vi "Func-엑셀 데이터를 그래프로 출력.vi"() -> ()   [LabVIEW 2015] (continued)
-40\t-39.51\t-24.372\n-40\t-39.51\t-24.377\n-40\t-39.51\t-24.385\n-40\t-39.52\t-24.391\n-40\t-39.52\t-24.396\n-40\t-39.53\t-24.404\n-40\t-39.54\t-24.406\n-40\t-39.54\t-24.41\n-40\t-39.55\t-24.416\n-40\t-39.55\t-24.418\n-40\t-39.56\t-24.424\n-40\t-39.57\t-24.428\n-40\t-39.57\t-24.436\n-40\t-39.58\t-24.442\n-40\t-39.58\t-24.446\n-40\t-39.58\t-24.453\n-40\t-39.58\t-24.456\n-40\t-39.58\t-24.461\n-40\t-39.59\t-24.466\n-40\t-39.59\t-24.471\n-40\t-39.59\t-24.475\n-40\t-39.6\t-24.478\n-40\t-39.6\t-24.486\n-40\t-39.61\t-24.495\n-40\t-39.61\t-24.5\n-40\t-39.62\t-24.504\n-40\t-39.62\t-24.512\n-40\t-39.62\t-24.522\n-40\t-39.63\t-24.521\n-40\t-39.63\t-24.529\n-40\t-39.63\t-24.535\n-40\t-39.63\t-24.539\n-40\t-39.64\t-24.548\n-40\t-39.64\t-24.549\n-40\t-39.64\t-24.556\n-40\t-39.65\t-24.557\n-40\t-39.65\t-24.566\n-40\t-39.65\t-24.573\n-40\t-39.65\t-24.576\n-40\t-39.66\t-24.585\n-40\t-39.66\t-24.593\n-40\t-39.67\t-24.597\n-40\t-39.67\t-24.602\n-40\t-39.68\t-24.609\n-40\t-39.68\t-24.614\n-40\t-39.68\t-24.618\n-40\t-39.69\t-24.62\n-40\t-39.69\t-24.628\n-40\t-39.69\t-24.633\n-40\t-39.7\t-24.636\n-40\t-39.7\t-24.643\n-40\t-39.71\t-24.652\n-40\t-39.71\t-24.66\n-40\t-39.71\t-24.667\n-40\t-39.71\t-24.672\n-40\t-39.71\t-24.676\n-40\t-39.72\t-24.682\n-40\t-39.72\t-24.684\n-40\t-39.72\t-24.687\n-40\t-39.72\t-24.691\n-40\t-39.72\t-24.693\n-40\t-39.72\t-24.699\n-40\t-39.72\t-24.705\n-40\t-39.72\t-24.714\n-40\t-39.73\t-24.719\n-40\t-39.73\t-24.729\n-40\t-39.73\t-24.737\n-40\t-39.73\t-24.744\n-40\t-39.74\t-24.747\n-40\t-39.74\t-24.753\n-40\t-39.74\t-24.76\n-40\t-39.74\t-24.764\n-40\t-39.74\t-24.769\n-40\t-39.74\t-24.772\n-40\t-39.74\t-24.78\n-40\t-39.75\t-24.784\n-40\t-39.75\t-24.787\n-40\t-39.75\t-24.795\n-40\t-39.75\t-24.796\n-40\t-39.76\t-24.802\n-40\t-39.76\t-24.807\n-40\t-39.76\t-24.812\n-40\t-39.76\t-24.818\n-40\t-39.76\t-24.822\n-40\t-39.76\t-24.828\n-40\t-39.77\t-24.832\n-40\t-39.77\t-24.839\n-40\t-39.78\t-24.842\n-40\t-39.78\t-24.845\n-40\t-39.78\t-24.857\n-40\t-39.78\t-24.864\n-40\t-39.79\t-24.87\n-40\t-39.79\t-24.879\n-40\t-39.79\t-24.888\n-40\t-39.79\t-24.893\n-40\t-39.8\t-24.896\n-40\t-39.8\t-24.9\n-40\t-39.8\t-24.903\n-40\t-39.8\t-24.908\n-40\t-39.81\t-24.909\n-40\t-39.81\t-24.915\n-40\t-39.81\t-24.923\n-40\t-39.81\t-24.926\n-40\t-39.81\t-24.93\n-40\t-39.81\t-24.937\n-40\t-39.81\t-24.944\n-40\t-39.81\t-24.948\n-40\t-39.82\t-24.954\n-40\t-39.82\t-24.962\n-40\t-39.82\t-24.967\n-40\t-39.83\t-24.972\n-40\t-39.83\t-24.974\n-40\t-39.83\t-24.979\n-40\t-39.83\t-24.985\n-40\t-39.84\t-24.986\n-40\t-39.84\t-24.995\n-40\t-39.84\t-25.003\n-40\t-39.84\t-25.011\n-40\t-39.84\t-25.014\n-40\t-39.85\t-25.022\n-40\t-39.85\t-25.029\n-40\t-39.85\t-25.031\n-40\t-39.86\t-25.034\n-40\t-39.86\t-25.039\n-40\t-39.86\t-25.044\n-40\t-39.86\t-25.049\n-40\t-39.87\t-25.054\n-40\t-39.87\t-25.059\n-40\t-39.87\t-25.067\n-40\t-39.87\t-25.069\n-40\t-39.88\t-25.077\n-40\t-39.88\t-25.082\n-40\t-39.88\t-25.088\n-40\t-39.88\t-25.093\n-40\t-39.88\t-25.1\n-40\t-39.88\t-25.106\n-40\t-39.88\t-25.11\n-40\t-39.88\t-25.116\n-40\t-39.88\t-25.121\n-40\t-39.88\t-25.126\n-40\t-39.88\t-25.134\n-40\t-39.88\t-25.138\n-40\t-39.89\t-25.145\n-40\t-39.89\t-25.154\n-40\t-39.89\t-25.161\n-40\t-39.89\t-25.163\n-40\t-39.9\t-25.168\n-40\t-39.9\t-25.172\n-40\t-39.9\t-25.176\n-40\t-39.9\t-25.181\n-40\t-39.9\t-25.186\n-40\t-39.9\t-25.194\n-40\t-39.91\t-25.2\n-40\t-39.91\t-25.207\n-40\t-39.92\t-25.212\n-40\t-39.92\t-25.219\n-40\t-39.92\t-25.223\n-40\t-39.92\t-25.227\n-40\t-39.93\t-25.236\n-40\t-39.93\t-25.239\n-40\t-39.93\t-25.246\n-40\t-39.93\t-25.253\n-40\t-39.93\t-25.258\n-40\t-39.94\t-25.263\n-40\t-39.94\t-25.267\n-40\t-39.94\t-25.274\n-40\t-39.95\t-25.279\n-40\t-39.95\t-25.285\n-40\t-39.95\t-25.29\n-40\t-39.95\t-25.295\n-40\t-39.95\t-25.3\n-40\t-39.95\t-25.305\n-40\t-39.95\t-25.311\n-40\t-39.95\t-25.316\n-40\t-39.96\t-25.32\n-40\t-39.96\t-25.321\n-40\t-39.96\t-25.326\n-40\t-39.97\t-25.328\n-40\t-39.97\t-25.331\n-40\t-39.97\t-25.338\n-40\t-39.97\t-25.344\n-40\t-39.97\t-25.35\n-40\t-39.97\t-25.36\n-40\t-39.97\t-25.363\n-40\t-39.98\t-25.364\n-40\t-39.98\t-25.367\n-40\t-39.98\t-25.37\n-40\t-39.98\t-25.373\n-40\t-39.98\t-25.379\n-40\t-39.98\t-25.389\n-40\t-39.98\t-25.398\n-40\t-39.98\t-25.408\n-40\t-39.98\t-25.413\n-40\t-39.99\t-25.418\n-40\t-39.99\t-25.424\n-40\t-40\t-25.425\n-40\t-40\t-25.428\n-40\t-40\t-25.432\n-40\t-40\t-25.437\n-40\t-40\t-25.445\n-40\t-40\t-25.453\n-40\t-40\t-25.458\n-40\t-40\t-25.461\n-40\t-40\t-25.47\n-40\t-40\t-25.477\n-40\t-40\t-25.48\n-40\t-40\t-25.486\n-40\t-40\t-25.492\n-40\t-40\t-25.498\n-40\t-40\t-25.501\n-40\t-40\t-25.504\n-40\t-40\t-25.507\n-40\t-40\t-25.509\n-40\t-40\t-25.512\n-40\t-40\t-25.517\n-40\t-40\t-25.522\n-40\t-40\t-25.525\n-40\t-40\t-25.53\n-40\t-40\t-25.539\n-40\t-40\t-25.545\n-40\t-40\t-25.549\n-40\t-40\t-25.557\n-40\t-40\t-25.563\n-40\t-40\t-25.568\n-40\t-40\t-25.572\n-40\t-40\t-25.579\n-40\t-40\t-25.583\n-40\t-40\t-25.589\n-40\t-40\t-25.594\n-40\t-40\t-25.596\n-40\t-40\t-25.603\n-40\t-40\t-25.605\n-40\t-40\t-25.61\n-40\t-40\t-25.618\n-40\t-40\t-25.62\n-40\t-40\t-25.626\n-40\t-40\t-25.631\n-40\t-40\t-25.638\n-40\t-40\t-25.645\n-40\t-40\t-25.648\n-40\t-40\t-25.655\n-40\t-40\t-25.661\n-40\t-40\t-25.667\n-40\t-40\t-25.671\n-40\t-40\t-25.677\n-40\t-40\t-25.682\n-40\t-40\t-25.687\n-40\t-40\t-25.691\n-40\t-40\t-25.697\n-40\t-40\t-25.698\n-40\t-40\t-25.704\n-40\t-40\t-25.707\n-40\t-40\t-25.711\n-40\t-40\t-25.716\n-40\t-40\t-25.723\n-40\t-40\t-25.731\n-40\t-40\t-25.736\n-40\t-40\t-25.742\n-40\t-40\t-25.746\n-40\t-40\t-25.749\n-40\t-40\t-25.754\n-40\t-40\t-25.758\n-40\t-40\t-25.764\n-40\t-40\t-25.769\n-40\t-40\t-25.775\n-40\t-40\t-25.784\n-40\t-40\t-25.791\n-40\t-40\t-25.793\n-40\t-40.02\t-25.802\n-40\t-40.02\t-25.808\n-40\t-40.02\t-25.814\n-40\t-40.02\t-25.816\n-40\t-40.02\t-25.82\n-40\t-40.02\t-25.825\n-40\t-40.02\t-25.828\n-40\t-40.02\t-25.835\n-40\t-40.02\t-25.837\n-40\t-40.02\t-25.846\n-40\t-40.02\t-25.85\n-40\t-40.02\t-25.854\n-40\t-40.02\t-25.865\n-40\t-40.02\t-25.867\n-40\t-40.02\t-25.867\n-40\t-40.02\t-25.873\n-40\t-40.02\t-25.879\n-40\t-40.02\t-25.885\n-40\t-40.02\t-25.887\n-40\t-40.02\t-25.891\n-40\t-40.02\t-25.898\n-40\t-40.02\t-25.902\n-40\t-40.02\t-25.904\n-40\t-40.02\t-25.904\n-40\t-40.02\t-25.912\n-40\t-40.02\t-25.916\n-40\t-40.02\t-25.92\n-40\t-40.02\t-25.927\n-40\t-40.02\t-25.934\n-40\t-40.02\t-25.942\n-40\t-40.02\t-25.949\n-40\t-40.02\t-25.951\n-40\t-40.02\t-25.952\n-40\t-40.02\t-25.956\n-40\t-40.02\t-25.961\n-40\t-40.02\t-25.963\n-40\t-40.02\t-25.965\n-40\t-40.02\t-25.972\n-40\t-40.02\t-25.982\n-40\t-40.02\t-25.99\n-40\t-40.02\t-25.993\n-40\t-40.02\t-25.997\n-40\t-40.02\t-26.003\n-40\t-40.02\t-26.008\n-40\t-40.02\t-26.016\n-40\t-40.02\t-26.021\n-40\t-40.02\t-26.029\n-40\t-40.02\t-26.034\n-40\t-40.02\t-26.039\n-40\t-40.02\t-26.043\n-40\t-40.02\t-26.042\n-40\t-40.02\t-26.049\n-40\t-40.02\t-26.05\n-40\t-40.02\t-26.053\n-40\t-40.02\t-26.062\n-40\t-40.02\t-26.067\n-40\t-40.02\t-26.072\n-40\t-40.02\t-26.075\n-40\t-40.02\t-26.079\n-40\t-40.02\t-26.083\n-40\t-40.02\t-26.089\n-40\t-40.02\t-26.093\n-40\t-40.02\t-26.098\n-40\t-40.02\t-26.106\n-40\t-40.02\t-26.109\n-40\t-40.02\t-26.117\n-40\t-40.02\t-26.123\n-40\t-40.02\t-26.126\n-40\t-40.02\t-26.13\n-40\t-40.02\t-26.135\n-40\t-40.02\t-26.14\n-40\t-40.02\t-26.142\n-40\t-40.03\t-26.145\n-40\t-40.03\t-26.152\n-40\t-40.03\t-26.157\n-40\t-40.03\t-26.163\n-40\t-40.03\t-26.167\n-40\t-40.03\t-26.173\n-40\t-40.03\t-26.181\n-40\t-40.03\t-26.184\n-40\t-40.03\t-26.188\n-40\t-40.03\t-26.192\n-40\t-40.03\t-26.194\n-40\t-40.03\t-26.195\n-40\t-40.03\t-26.202\n-40\t-40.02\t-26.207\n-40\t-40.02\t-26.211\n-40\t-40.02\t-26.219\n-40\t-40.02\t-26.227\n-40\t-40.02\t-26.231\n-40\t-40.02\t-26.236\n-40\t-40.02\t-26.239\n-40\t-40.02\t-26.242\n-40\t-40.02\t-26.248\n-40\t-40.02\t-26.25\n-40\t-40.02\t-26.256\n-40\t-40.02\t-26.266\n-40\t-40.02\t-26.271\n-40\t-40.02\t-26.277\n-40\t-40.02\t-26.28\n-40\t-40.02\t-26.286\n-40\t-40.02\t-26.29\n-40\t-40.02\t-26.292\n-40\t-40.02\t-26.295\n-40\t-40.02\t-26.298\n-40\t-40.02\t-26.307\n-40\t-40.02\t-26.312\n-40\t-40.02\t-26.32\n-40\t-40.02\t-26.327\n-40\t-40.02\t-26.334\n-40\t-40.03\t-26.337\n-40\t-40.03\t-26.343\n-40\t-40.03\t-26.347\n-40\t-40.03\t-26.349\n-40\t-40.03\t-26.354\n-40\t-40.03\t-26.356\n-40\t-40.03\t-26.362\n-40\t-40.03\t-26.368\n-40\t-40.03\t-26.371\n-40\t-40.03\t-26.375\n-40\t-40.03\t-26.381\n-40\t-40.03\t-26.387\n-40\t-40.03\t-26.39\n-40\t-40.03\t-26.396\n-40\t-40.03\t-26.402\n-40\t-40.02\t-26.407\n-40\t-40.02\t-26.41\n-40\t-40.02\t-26.413\n-40\t-40.02\t-26.418\n-40\t-40.02\t-26.42\n-40\t-40.02\t-26.423\n-40\t-40.02\t-26.426\n-40\t-40.02\t-26.436\n-40\t-40.02\t-26.439\n-40\t-40.02\t-26.445\n-40\t-40.02\t-26.453\n-40\t-40.02\t-26.455\n-40\t-40.02\t-26.46\n-40\t-40.02\t-26.461\n-40\t-40.02\t-26.469\n-40\t-40.02\t-26.47\n-40\t-40.02\t-26.477\n-40\t-40.02\t-26.482\n-40\t-40.02\t-26.49\n-40\t-40.02\t-26.497\n-40\t-40.02\t-26.5\n-40\t-40.02\t-26.506\n-40\t-40.02\t-26.511\n-40\t-40.02\t-26.52\n-40\t-40.02\t-26.521\n-40\t-40.02\t-26.527\n-40\t-40.02\t-26.532\n-40\t-40.02\t-26.536\n-40\t-40.02\t-26.538\n-40\t-40.02\t-26.542\n-40\t-40.02\t-26.546\n-40\t-40.02\t-26.555\n-40\t-40.02\t-26.558\n-40\t-40.02\t-26.564\n-40\t-40.02\t-26.57\n-40\t-40.02\t-26.573\n-40\t-40.02\t-26.578\n-40\t-40.02\t-26.582\n-40\t-40.02\t-26.584\n-40\t-40.02\t-26.588\n-40\t-40.02\t-26.594\n-40\t-40.02\t-26.595\n-40\t-40.02\t-26.594\n-40\t-40.02\t-26.598\n-40\t-40.02\t-26.607\n-40\t-40.02\t-26.609\n-40\t-40.02\t-26.613\n-40\t-40.02\t-26.62\n-40\t-40.02\t-26.627\n-40\t-40.02\t-26.63\n-40\t-40.02\t-26.634\n-40\t-40.02\t-26.637\n-40\t-40.02\t-26.645\n-40\t-40.02\t-26.646\n-40\t-40.02\t-26.651\n-40\t-40.02\t-26.658\n-40\t-40.02\t-26.66\n-40\t-40.02\t-26.664\n-40\t-40\t-26.67\n-40\t-40\t-26.675\n-40\t-40\t-26.677\n-40\t-40\t-26.684\n-40\t-40\t-26.687\n-40\t-40\t-26.693\n-40\t-40\t-26.696\n-40\t-40\t-26.7\n-40\t-40\t-26.708\n-40\t-40\t-26.711\n-40\t-40\t-26.713\n-40\t-40\t-26.716\n-40\t-40.02\t-26.72\n-40\t-40\t-26.725\n-40\t-40\t-26.725\n-40\t-40\t-26.732\n-40\t-40\t-26.739\n-40\t-40\t-26.743\n-40\t-40.02\t-26.751\n-40\t-40.02\t-26.755\n-40\t-40.02\t-26.763\n-40\t-40.02\t-26.768\n-40\t-40.02\t-26.771\n-40\t-40\t-26.774\n-40\t-40.02\t-26.776\n-40\t-40.02\t-26.78\n-40\t-40.02\t-26.782\n-40\t-40.02\t-26.786\n-40\t-40.02\t-26.789\n-40\t-40.02\t-26.795\n-40\t-40.02\t-26.801\n-40\t-40.02\t-26.802\n-40\t-40.02\t-26.805\n-40\t-40.02\t-26.808\n-40\t-40.02\t-26.811\n-40\t-40.02\t-26.815\n-40\t-40.02\t-26.823\n-40\t-40.02\t-26.829\n-40\t-40.02\t-26.833\n-40\t-40.02\t-26.84\n-40\t-40.02\t-26.848\n-40\t-40.02\t-26.847\n-40\t-40.02\t-26.852\n-40\t-40.02\t-26.856\n-40\t-40.02\t-26.861\n-40\t-40.02\t-26.863\n-40\t-40.02\t-26.866\n-40\t-40.02\t-26.873\n-40\t-40.02\t-26.88\n-40\t-40.02\t-26.883\n-40\t-40.02\t-26.888\n-40\t-40.02\t-26.891\n-40\t-40.02\t-26.894\n-40\t-40.02\t-26.899\n-40\t-40.02\t-26.9\n-40\t-40.02\t-26.903\n-40\t-40.02\t-26.909\n-40\t-40.02\t-26.914\n-40\t-40.02\t-26.918\n-40\t-40.02\t-26.924\n-40\t-40.02\t-26.929\n-40\t-40.02\t-26.932\n-40\t-40.02\t-26.938\n-40\t-40.02\t-26.944\n-40\t-40.02\t-26.946\n-40\t-40.02\t-26.949\n-40\t-40.02\t-26.95\n-40\t-40.02\t-26.955\n-40\t-40.02\t-26.958\n-40\t-40.02\t-26.959\n-40\t-40.02\t-26.965\n-40\t-40.02\t-26.971\n-40\t-40.02\t-26.977\n-40\t-40.02\t-26.983\n-40\t-40.02\t-26.99\n-40\t-40.02\t-26.993\n-40\t-40.02\t-26.996\n-40\t-40.02\t-27.003\n-40\t-40.02\t-27.006\n-40\t-40.02\t-27.011\n-40\t-40.02\t-27.013\n-40\t-40.02\t-27.017\n-40\t-40.02\t-27.019\n-40\t-40.02\t-27.025\n-40\t-40.02\t-27.028\n-40\t-40.02\t-27.027\n-40\t-40.02\t-27.03\n-40\t-40.02\t-27.036\n-40\t-40.02\t-27.041\n-40\t-40.02\t-27.041\n-40\t-40.02\t-27.046\n-40\t-40.02\t-27.052\n-40\t-40.02\t-27.062\n-40\t-40.02\t-27.063\n-40\t-40.02\t-27.068\n-40\t-40.02\t-27.077\n-40\t-40.02\t-27.08\n-40\t-40.02\t-27.084\n-40\t-40.02\t-27.083\n-40\t-40.02\t-27.084\n-40\t-40.02\t-27.085\n-40\t-40.02\t-27.092\n-40\t-40.02\t-27.096\n-40\t-40.02\t-27.096\n-40\t-40.02\t-27.103\n-40\t-40.02\t-27.112\n-40\t-40.02\t-27.118\n-40\t-40.02\t-27.121\n-40\t-40.02\t-27.127\n-40\t-40.02\t-27.131\n-40\t-40.02\t-27.137\n-40\t-40.02\t-27.139\n-40\t-40.02\t-27.141\n-40\t-40.02\t-27.143\n-40\t-40.02\t-27.144\n-40\t-40.02\t-27.147\n-40\t-40.02\t-27.153\n-40\t-40.02\t-27.157\n-40\t-40.02\t-27.158\n-40\t-40.02\t-27.166\n-40\t-40.02\t-27.171\n-40\t-40.02\t-27.172\n-40\t-40.02\t-27.174\n-40\t-40.02\t-27.176\n-40\t-40.02\t-27.181\n-40\t-40.02\t-27.187\n-40\t-40.02\t-27.187\n-40\t-40.02\t-27.193\n-40\t-40.02\t-27.198\n-40\t-40.02\t-27.2\n-40\t-40\t-27.205\n-40\t-40\t-27.209\n-40\t-40\t-27.216\n-40\t-40\t-27.221\n-40\t-40\t-27.226\n-40\t-40\t-27.229\n-40\t-40\t-27.23\n-40\t-40\t-27.233\n-40\t-40\t-27.234\n-40\t-40\t-27.238\n-40\t-40\t-27.245\n-40\t-40\t-27.25\n-40\t-40\t-27.254\n-40\t-40\t-27.261\n-40\t-40\t-27.264\n-40\t-40\t-27.267\n-40\t-40\t-27.268\n-40\t-40\t-27.272\n-40\t-40\t-27.277\n-40\t-40\t-27.28\n-40\t-40\t-27.283\n-40\t-40\t-27.287\n-40\t-40\t-27.29\n-40\t-40\t-27.291\n-40\t-40\t-27.296\n-40\t-40\t-27.3\n-40\t-40\t-27.305\n-40\t-40\t-27.309\n-40\t-40\t-27.316\n-40\t-40\t-27.321\n-40\t-40\t-27.321\n-40\t-40\t-27.321\n-40\t-40\t-27.322\n-40\t-40\t-27.327\n-40\t-40\t-27.329\n-40\t-40\t-27.333\n-40\t-40\t-27.339\n-40\t-40\t-27.348\n-40\t-40\t-27.352\n-40\t-40\t-27.355\n-40\t-40\t-27.358\n-40\t-40\t-27.361\n-40\t-40\t-27.364\n-40\t-40\t-27.368\n-40\t-40\t-27.37\n-40\t-40\t-27.371\n-40\t-40\t-27.379\n-40\t-40\t-27.382\n-40\t-40\t-27.384\n-40\t-40\t-27.387\n-40\t-40\t-27.393\n-40\t-40\t-27.394\n-40\t-40\t-27.395\n-40\t-40\t-27.398\n-40\t-40\t-27.401\n-40\t-40\t-27.406\n-40\t-40\t-27.409\n-40\t-40\t-27.415\n-40\t-40\t-27.418\n-40\t-40\t-27.42\n-40\t-40\t-27.425\n-40\t-40\t-27.429\n-40\t-40\t-27.432\n-40\t-40\t-27.437\n-40\t-40\t-27.445\n-40\t-40\t-27.451\n-40\t-40\t-27.454\n-40\t-40\t-27.454\n-40\t-40\t-27.455\n-40\t-40\t-27.457\n-40\t-40\t-27.461\n-40\t-40\t-27.462\n-40\t-40\t-27.465\n-40\t-40\t-27.474\n-40\t-40\t-27.478\n-40\t-40\t-27.484\n-40\t-40\t-27.491\n-40\t-40\t-27.494\n-40\t-40\t-27.499\n-40\t-40\t-27.5\n-40\t-40\t-27.501\n-40\t-40\t-27.502\n-40\t-40\t-27.503\n-40\t-40\t-27.506\n-40\t-40\t-27.507\n-40\t-40\t-27.508\n-40\t-40\t-27.512\n-40\t-40\t-27.515\n-40\t-40\t-27.521\n-40\t-40\t-27.523\n-40\t-40\t-27.527\n-40\t-40\t-27.539\n-40\t-40\t-27.545\n-40\t-40\t-27.549\n-40\t-40\t-27.551\n-40\t-40\t-27.556\n-40\t-40\t-27.561\n-40\t-40\t-27.563\n-40\t-40\t-27.567\n-40\t-40\t-27.571\n-40\t-40\t-27.572\n-40\t-40\t-27.575\n-40\t-40\t-27.58\n-40\t-40\t-27.585\n-40\t-40\t-27.587\n-40\t-40\t-27.588\n-40\t-40\t-27.593\n-40\t-40\t-27.595\n-40\t-40\t-27.595\n-40\t-40\t-27.598\n-40\t-40\t-27.602\n-40\t-40\t-27.608\n-40\t-40\t-27.612\n-40\t-40\t-27.616\n-40\t-40\t-27.619\n-40\t-40\t-27.624\n-40\t-40\t-27.627\n-40\t-40\t-27.629\n-40\t-40\t-27.634\n-40\t-40\t-27.636\n-40\t-40\t-27.636\n-40\t-40\t-27.641\n-40\t-40\t-27.647\n-40\t-40\t-27.65\n-40\t-40\t-27.655\n-40\t-40\t-27.656\n-40\t-40\t-27.66\n-40\t-40\t-27.661\n-40\t-40\t-27.657\n-40\t-40\t-27.658\n-40\t-40\t-27.664\n-40\t-40\t-27.67\n-40\t-40\t-27.675\n-40\t-40\t-27.677\n-40\t-40\t-27.681\n-40\t-40\t-27.687\n-40\t-40\t-27.686\n-40\t-40\t-27.686\n-40\t-40\t-27.689\n-40\t-40\t-27.693\n-40\t-40\t-27.697\n-40\t-40\t-27.701\n-40\t-40\t-27.708\n-40\t-40\t-27.712\n-40\t-40\t-27.714\n-40\t-40\t-27.721\n-40\t-40\t-27.725\n-40\t-40\t-27.726\n-40\t-40\t-27.727\n-40\t-40\t-27.731\n-40\t-40\t-27.73\n-40\t-40\t-27.73\n-40\t-40\t-27.736\n-40\t-40\t-27.736\n-40\t-40\t-27.745\n-40\t-40\t-27.748\n-40\t-40\t-27.753\n-40\t-40\t-27.761\n-40\t-40\t-27.761\n-40\t-40\t-27.766\n-40\t-40\t-27.765\n-40\t-40\t-27.77\n-40\t-40\t-27.773\n-40\t-40\t-27.779\n-40\t-40\t-27.782\n-40\t-40\t-27.783\n-40\t-40\t-27.789\n-40\t-40\t-27.791\n-40\t-40\t-27.792\n-40\t-40\t-27.793\n-40\t-40\t-27.796\n-40\t-40\t-27.803\n-40\t-40\t-27.806\n-40\t-40\t-27.809\n-40\t-40\t-27.816\n-40\t-40\t-27.82\n-40\t-40\t-27.822\n-40\t-40\t-27.824\n-40\t-40\t-27.827\n-40\t-40\t-27.83\n-40\t-40\t-27.832\n-40\t-40\t-27.834\n-40\t-40\t-27.837\n-40\t-40\t-27.84\n-40\t-40\t-27.845\n-40\t-40\t-27.846\n-40\t-40\t-27.849\n-40\t-40\t-27.852\n-40\t-40\t-27.854\n-40\t-40\t-27.855\n-40\t-40\t-27.857\n-40\t-40\t-27.864\n-40\t-40\t-27.869\n-40\t-40\t-27.87\n-40\t-40\t-27.871\n-40\t-40\t-27.876\n-40\t-40\t-27.879\n-40\t-40\t-27.879\n-40\t-40\t-27.88\n-40\t-40\t-27.884\n-40\t-40\t-27.887\n-40\t-40\t-27.893\n-40\t-40\t-27.896\n-40\t-40\t-27.9\n-40\t-40\t-27.905\n-40\t-40\t-27.904\n-40\t-40\t-27.909\n-40\t-40\t-27.909\n-40\t-40\t-27.908\n-40\t-40\t-27.909\n-40\t-40\t-27.91\n-40\t-40\t-27.919\n-40\t-40\t-27.922\n-40\t-40\t-27.93\n-40\t-40\t-27.937\n-40\t-40\t-27.939\n-40\t-40\t-27.943\n-40\t-40\t-27.943\n-40\t-40\t-27.945\n-40\t-40\t-27.946\n-40\t-40\t-27.946\n-40\t-40\t-27.947\n-40\t-40\t-27.952\n-40\t-40\t-27.955\n-40\t-40\t-27.958\n-40\t-40\t-27.961\n-40\t-40\t-27.965\n-40\t-40\t-27.97\n-40\t-40\t-27.973\n-40\t-40\t-27.975\n-40\t-40\t-27.975\n-40\t-40\t-27.979\n-40\t-40\t-27.98\n-40\t-40\t-27.985\n-40\t-40\t-27.989\n-40\t-40\t-27.992\n-40\t-40\t-27.994\n-40\t-40\t-28.001\n-40\t-40\t-28.005\n-40\t-40\t-28.005\n-40\t-40\t-28.004\n-40\t-40\t-28.008\n-40\t-40\t-28.013\n-40\t-40\t-28.014\n-40\t-40\t-28.016\n-40\t-40\t-28.019\n-40\t-40\t-28.027\n-40\t-40\t-28.03\n-40\t-40\t-28.032\n-40\t-40\t-28.038\n-40\t-40\t-28.042\n-40\t-40\t-28.041\n-40\t-40\t-28.043\n-40\t-40\t-28.04\n-40\t-40\t-28.044\n-40\t-40\t-28.041\n-40\t-40\t-28.046\n-40\t-40\t-28.05\n-40\t-40\t-28.053\n-40\t-40\t-28.057\n-40\t-40\t-28.059\n-40\t-40\t-28.064\n-40\t-40\t-28.066\n-40\t-40\t-28.07\n-40\t-40\t-28.078\n-40\t-40\t-28.079\n-40\t-40\t-28.083\n-40\t-40\t-28.083\n-40\t-40\t-28.085\n-40\t-40\t-28.086\n-40\t-40\t-28.086\n-40\t-40\t-28.093\n-40\t-40\t-28.093\n-40\t-40\t-28.1\n-40\t-40\t-28.099\n-40\t-40\t-28.104\n-40\t-40\t-28.105\n-40\t-40\t-28.107\n-40\t-40\t-28.112\n-40\t-40\t-28.118\n-40\t-40\t-28.125\n-40\t-40\t-28.124\n-40\t-40\t-28.129\n-40\t-40\t-28.128\n-40\t-40\t-28.129\n-40\t-40\t-28.128\n-40\t-40\t-28.127\n-40\t-40\t-28.13\n-40\t-40\t-28.134\n-40\t-40\t-28.139\n-40\t-40\t-28.143\n-40\t-40\t-28.145\n-40\t-40\t-28.148\n-40\t-40\t-28.152\n-40\t-40\t-28.155\n-40\t-40\t-28.158\n-40\t-40\t-28.159\n-40\t-40\t-28.164\n-40\t-40\t-28.166\n-40\t-40\t-28.169\n-40\t-40\t-28.171\n-40\t-40\t-28.171\n-40\t-40\t-28.173\n-40\t-40\t-28.176\n-40\t-40\t-28.178\n-40\t-40\t-28.179\n-40\t-40\t-28.18\n-40\t-40\t-28.181\n-40\t-40\t-28.183\n-40\t-40\t-28.189\n-40\t-40\t-28.19\n-40\t-40\t-28.195\n-40\t-40\t-28.198\n-40\t-40\t-28.205\n-40\t-40\t-28.207\n-40\t-40\t-28.205\n-40\t-40\t-28.21\n-40\t-40\t-28.212\n-40\t-40\t-28.216\n-40\t-40\t-28.214\n-40\t-40\t-28.221\n-40\t-40\t-28.226\n-40\t-40\t-28.223\n-40\t-40\t-28.227\n-40\t-40\t-28.228\n-40\t-40\t-28.231\n-40\t-40\t-28.232\n-40\t-40\t-28.232\n-40\t-40\t-28.236\n-40\t-40\t-28.237\n-40\t-40\t-28.238\n-40\t-40\t-28.241\n-40\t-40\t-28.246\n-40\t-40\t-28.25\n-40\t-40\t-28.258\n-40\t-40\t-28.262\n-40\t-40\t-28.266\n-40\t-40\t-28.267\n-40\t-40\t-28.268\n-40\t-40\t-28.27\n-40\t-40\t-28.267\n-40\t-40\t-28.27\n-40\t-40\t-28.271\n-40\t-40\t-28.279\n-40\t-40\t-28.28\n-40\t-40\t-28.284\n-40\t-40\t-28.289\n-40\t-40\t-28.289\n-40\t-40\t-28.289\n-40\t-40\t-28.289\n-40\t-40\t-28.293\n-40\t-40\t-28.293\n-40\t-40\t-28.294\n-40\t-40\t-28.3\n-40\t-40\t-28.304\n-40\t-40\t-28.306\n-40\t-40\t-28.311\n-40\t-40\t-28.313\n-40\t-40\t-28.317\n-40\t-40\t-28.32\n-40\t-40\t-28.324\n-40\t-40\t-28.325\n-40\t-40\t-28.329\n-40\t-40\t-28.332\n-40\t-40\t-28.332\n-40\t-40\t-28.337\n-40\t-40\t-28.334\n-40\t-40\t-28.337\n-40\t-40\t-28.339\n-40\t-40\t-28.339\n-40\t-40\t-28.343\n-40\t-40\t-28.339\n-40\t-40\t-28.344\n-40\t-40\t-28.343\n-40\t-40\t-28.344\n-40\t-40\t-28.349\n-40\t-40\t-28.35\n-40\t-40\t-28.355\n-40\t-40\t-28.355\n-40\t-40\t-28.359\n-40\t-40\t-28.364\n-40\t-40\t-28.363\n-40\t-40\t-28.364\n-40\t-40\t-28.37\n-40\t-40\t-28.376\n-40\t-40\t-28.38\n-40\t-40\t-28.381\n-40\t-40\t-28.384\n-40\t-40\t-28.388\n-40\t-40\t-28.388\n-40\t-40\t-28.389\n-40\t-40\t-28.39\n-40\t-40\t-28.394\n-40\t-40\t-28.397\n-40\t-40\t-28.398\n-40\t-40\t-28.404\n-40\t-40\t-28.406\n-40\t-40\t-28.408\n-40\t-40\t-28.41\n-40\t-40\t-28.414\n-40\t-40\t-28.417
